vi "Write Relative_.vi"(8 "error in (no error)":errorcluster, 10 "Relative?":bool, 11 "PathCommands in":refnum<class "PathCommands.lvclass">) -> (0 "error out":errorcluster, 3 "PathCommands out":refnum<class "PathCommands.lvclass">)   [LabVIEW 2019, in "PathCommands.lvclass"]
uses:
  PathCommands.lvclass
  PathCommands.lvclass/PathCommands.ctl
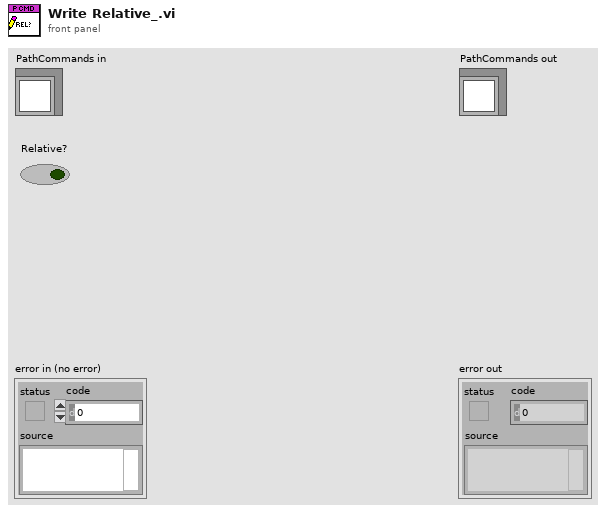
[diagram p1: front panel]
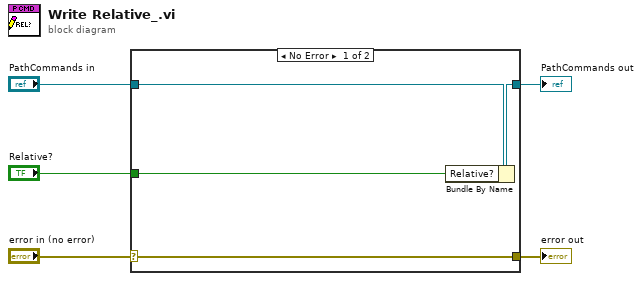
[diagram p0: block diagram]
diagram:
  n1 = case shown="No Error" "error in (no error)" {
    selector: "error in (no error)" -> [w9 w10]
    tunnel: [w9 w10] -> w4
    tunnel: [w7 w11] -> w2
    tunnel: "PathCommands in" -> [w8 w11]
    tunnel: "Relative?" -> [w6 _]
    frame No Error {
      n2 = Bundle By Name(cluster=w8, "Relative?"=w6) -> (w7:refnum<class "PathCommands.lvclass">)
    }
    frame Error {
    }
  }
  "error out" <- w4
  "PathCommands out" <- w2
